vi "Test Lookup Column.vi"() -> ()   [LabVIEW 2020, in "Test.lvlib"]
uses:
  Test.lvlib
  User/Values.ctl
  Conditum SQLite/SQLite/SQLite.lvclass
  C:/Program Files (x86)/National Instruments/LabVIEW 2020/vi.lib/IlluminatedG/IG Conditum/Conditum/Database Platform/Database Platform.lvclass
  User/User.lvclass
  C:/Program Files (x86)/National Instruments/LabVIEW 2020/vi.lib/IlluminatedG/IG Conditum/Conditum/Entity/Entity.lvclass
  <vilib>/IlluminatedG/IG Conditum/Conditum/Columns/Type/Type.lvclass/Type.ctl
  <vilib>/IlluminatedG/IG Conditum/Conditum/Columns/Text/Text.lvclass/Text.ctl
  <vilib>/IlluminatedG/IG Conditum/Conditum/Columns/String/String.lvclass/String.ctl
  User/User.lvclass/User.ctl
  <vilib>/IlluminatedG/IG Conditum/Conditum/Columns/Timestamp/Timestamp.lvclass/Timestamp.ctl
  <vilib>/IlluminatedG/IG Conditum/Conditum/Columns/Boolean/Boolean.lvclass/Boolean.ctl
  <vilib>/IlluminatedG/IG Conditum/Conditum/Columns/Integer/Integer.lvclass/Integer.ctl
  9994fd39-d4bd-4524-a1a0-d8ab6d697691.vi
  <vilib>/IlluminatedG/IG Conditum/Conditum/Columns/Text/Set.vi
  <vilib>/IlluminatedG/IG Conditum/Conditum/Columns/String/Set.vi
  <vilib>/IlluminatedG/IG Conditum/Conditum/Columns/Type/Type.vi
  <vilib>/IlluminatedG/IG Conditum/Conditum/Columns/String/Get.vi
  <vilib>/IlluminatedG/IG Conditum/Conditum/Columns/Timestamp/Get.vi
  <vilib>/IlluminatedG/IG Conditum/Conditum/Columns/Boolean/Get.vi
  <vilib>/IlluminatedG/IG Conditum/Conditum/Columns/Integer/Get.vi
  <vilib>/IlluminatedG/IG Conditum/Conditum/Columns/Type/Clear NULL.vi
  <vilib>/IlluminatedG/IG Conditum/Conditum/Columns/Text/Text.lvclass
  C:/Program Files (x86)/National Instruments/LabVIEW 2020/vi.lib/IlluminatedG/IG Conditum/Conditum/Columns/Type/Type.lvclass
  <vilib>/IlluminatedG/IG Conditum/Conditum/Columns/String/String.lvclass
  <vilib>/IlluminatedG/IG Conditum/Conditum/Entity Manager/Entity Column by Name.vi
  <vilib>/Utility/error.llb/Error Cluster From Error Code.vi
  <vilib>/IlluminatedG/IG Conditum/Conditum/Entity Manager/Find Entity by Type.vi
  <vilib>/IlluminatedG/IG Conditum/Conditum/Columns/Type/Type.lvclass
  <vilib>/IlluminatedG/IG Conditum/Conditum/Entity Manager/Entity Manager.lvclass
panel:
  in  "Username":string
  out "Values":T1
  out "error out":errorcluster
  in  "DB Path":path=path "C:/dev/lv20CE/lv-conditum-sqlite/Test/test.db"
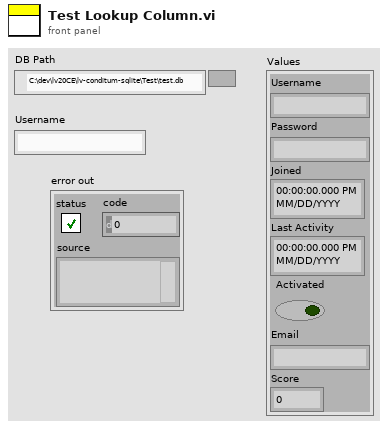
[diagram p1: front panel]
types:
  T1 = typedef "Test.lvlib/User.lvclass/Values.ctl" = cluster{"Username":string, "Password":string, "Joined":timestamp, "Last Activity":timestamp, "Activated":bool, "Email":string, "Score":i64}
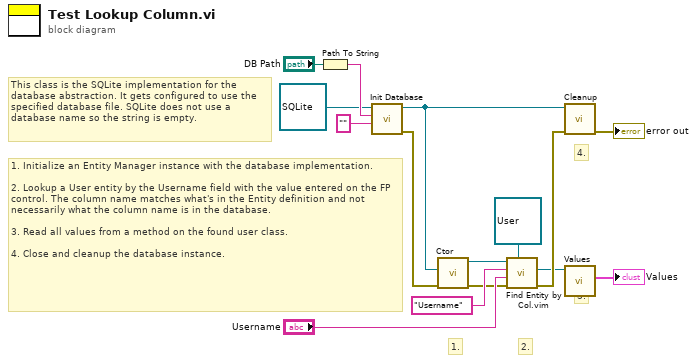
[diagram p0: block diagram]
diagram:
  # "1. Initialize an Entity Manager instance with the database implementation.\n\n2. Lookup a User entity by the Username field with the value entered on the FP control. The column name matches what's in the Entity definition and not necessarily what the column name is in the database.\n\n3. Read all values from a method on the found user class.\n\n4. Close and cleanup the database instance."
  # "4."
  # "3."
  # "2."
  # "1."
  # "This class is the SQLite implementation for the database abstraction. It gets configured to use the specified database file. SQLite does not use a database name so the string is empty."
  n1 = Path To String(path="DB Path") -> (string=w14:string)
  n2 = call-dynamic "Init Database.vi"("Database"="", "Resource"=w14, "Database in"=refnum<class "SQLite.lvclass"> refnum) -> ("error out"=w4:errorcluster, "Database out"=w3:refnum<class "SQLite.lvclass">)  [unwired: 7 in]
  n3 = call <vilib>:"Ctor.vi"("error in (no error)"=w4, "Database"=w3) -> ("error out"=w1:errorcluster, "Entity Manager out"=w2:refnum<class "Entity Manager.lvclass">)  [unwired: 8 in]
  n4 = call "Find Entity by Col.vim"("Entity Type"=refnum<class "User.lvclass"> refnum ("Test.lvlib:User.lvclass"), "error in (no error)"=w1, "Value"="Username", "Name"="Username", "Entity Manager in"=w2) -> ("error out"=w8:errorcluster, "Entity"=w7:refnum<class "User.lvclass">)  [unwired: 4 in, 1 out]
  n5 = call-dynamic "Cleanup.vi"("error in (no error)"=w8, "SQLite in"=w3) -> ("error out"=→"error out":errorcluster)  [unwired: 9 in]
  n6 = call "Values.vi"("User in"=w7) -> ("Values"=→"Values":T1)  [unwired: 10 in]
